vi "Read StandardWfrms.vi"(8 "error in (no error)":errorcluster, 11 "StandardFunction in":refnum<class "StandardFunction.lvclass">) -> (0 "error out":errorcluster, 2 "StandardWfrms":T1, 3 "StandardFunction out":refnum<class "StandardFunction.lvclass">)   [LabVIEW 2018, in "Functions.lvlib" / "StandardFunction.lvclass"]
uses:
  StandardFunction.lvclass
  TypeDefs/StdWfrms.ctl
  TypeDefs/StdWfrm.ctl
  StandardFunction.lvclass/StandardFunction.ctl
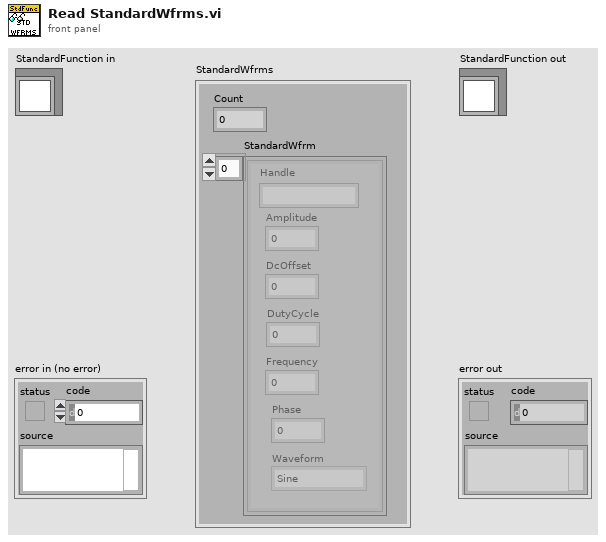
[diagram p1: front panel]
types:
  T1 = typedef "Functions.lvlib/StandardFunction.lvclass/StdWfrms.ctl" = cluster{"Count":u16, "StandardWfrm":T2[]}
  T2 = typedef "Functions.lvlib/StandardFunction.lvclass/StdWfrm.ctl" = cluster{"Amplitude":dbl, "DcOffset":dbl, "DutyCycle":dbl, "Frequency":dbl, "Phase":dbl, "Waveform":enum16{"Sine", "Square", "Triangle", "Ramp Up", "Ramp Down", "DC"}, "Handle":string}
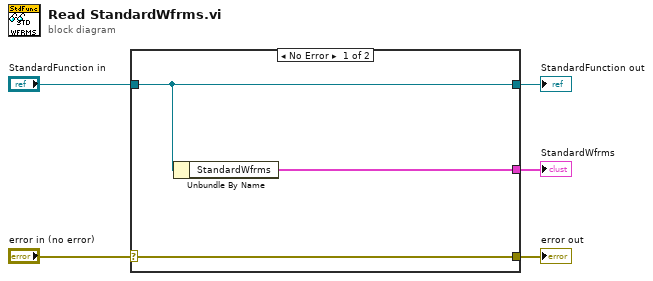
[diagram p0: block diagram]
diagram:
  n1 = case shown="No Error" "error in (no error)" {
    selector: "error in (no error)" -> [w8 w9]
    tunnel: [w8 w9] -> w4
    tunnel: [w7 w10] -> w2
    tunnel: "StandardFunction in" -> [w7 w10]
    tunnel: [w6 _] -> w1
    frame No Error {
      n2 = Unbundle By Name(w7) -> ("StandardWfrms"=w6:T1)
    }
    frame Error {
    }
  }
  "error out" <- w4
  "StandardFunction out" <- w2
  "StandardWfrms" <- w1
